vi "Get Logic Statuses.vi"(8 "error in (no error)":errorcluster, 11 "VacuumLine in":refnum<class "VacuumLine.lvclass">) -> (0 "error out":errorcluster, 1 "disconnected":bool, 2 "Array of Logic Statuses":T1(array[cluster]), 3 "VacuumLine out":refnum<class "VacuumLine.lvclass">)   [LabVIEW 2016, in "Hardware.lvlib" / "VacuumLine.lvlib" / "VacuumLine.lvclass"]
uses:
  <userlib>/Common Components/Hardware/Abstract System/VacuumLine/VacuumLine/VacuumLine.lvclass
  <userlib>/Common Components/Hardware/Abstract System/VacuumLine/VacuumLine/VacuumLine.lvclass/VacuumLine.ctl
  <userlib>/Common Components/Hardware/LogicIO/LogicIO/LogicIO.lvclass
  C:/Program Files (x86)/National Instruments/LabVIEW 2016/user.lib/Common Components/Hardware/Abstract Hardware/Hardware.lvclass
  <userlib>/Common Components/Hardware/LogicIO/LogicIO/Get Logic Status (multiple).vi
  <userlib>/Common Components/Hardware/Abstract Hardware/Hardware.lvclass
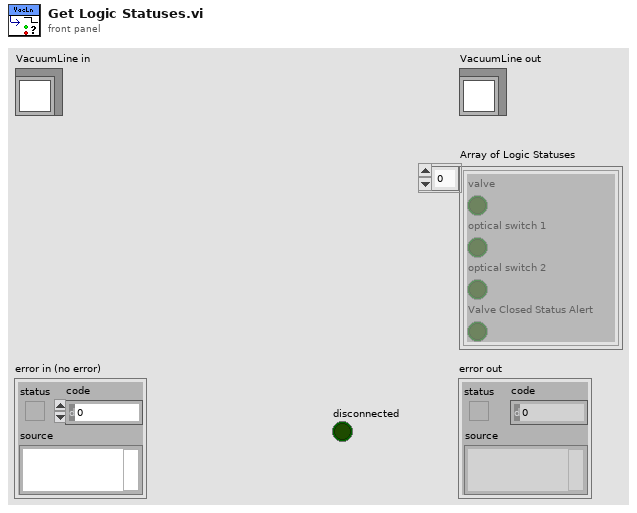
[diagram p1: front panel]
types:
  T1 = cluster{"valve":bool, "optical switch 1":bool, "optical switch 2":bool, "Valve Closed Status Alert":bool}[]
  T2 = cluster{"valve":bool, "optical switch -":bool, "optical switch +":bool, "Valve Closed Status Alert":bool}[]
  T3 = typedef "Hardware.lvlib/VacuumLine.lvlib/VacuumLine.lvclass/Valve Complex.ctl" = cluster{"LogicIO Module":string, "Valve Open":T4, "Optical Switch -":T4, "Optical Switch +":T4, "Valve Closed Status Alert":cluster{"Pin#":u8, "Option":enum16{"Not Used", "Normally Closed"}}}
  T4 = typedef "Hardware.lvlib/VacuumLine.lvlib/VacuumLine.lvclass/Logic Cluster.ctl" = cluster{"Pin#":u8, "Location":dbl, "Tolerance":dbl}
  T5 = cluster{"Array of Logic Statuses[0]":bool, "Array of Logic Statuses[1]":bool, "Array of Logic Statuses[2]":bool, "Array of Logic Statuses[3]":bool}
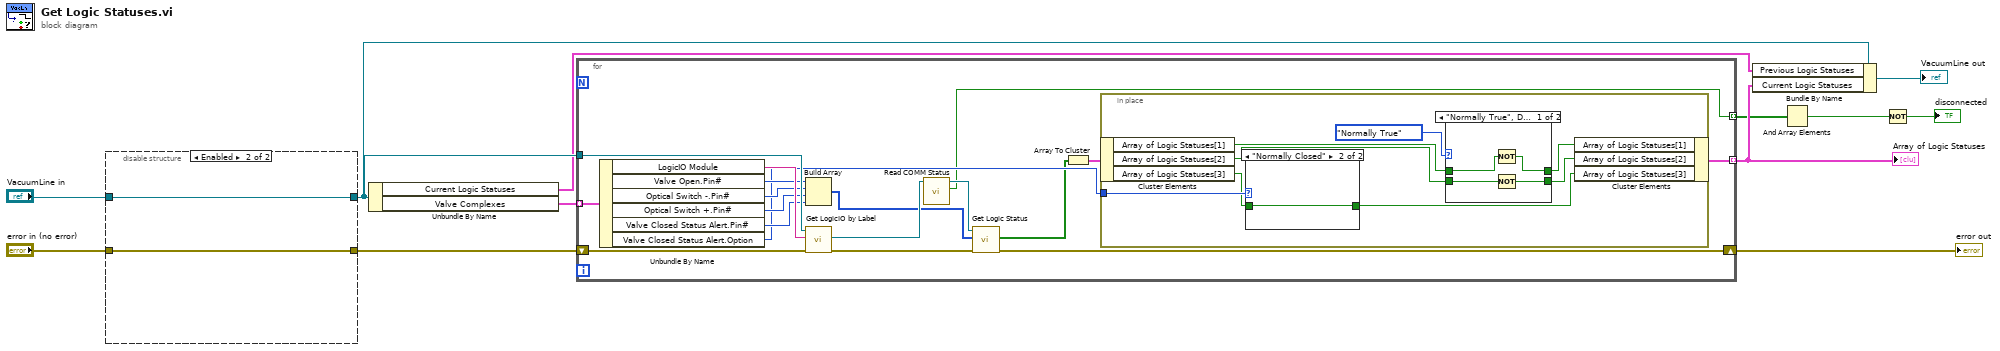
[diagram p0: block diagram]
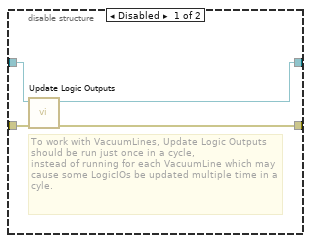
[diagram p2: hidden frame]
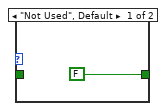
[diagram p3: hidden frame]
diagram:
  n1 = disable-structure shown="Enabled" {
    disable-tunnel: "error in (no error)" -> [w16 w17]
    disable-tunnel: [w15 w17] -> w9
    disable-tunnel: "VacuumLine in" -> [w14 w18]
    disable-tunnel: [w13 w18] -> w7
    frame Disabled {
      # "To work with VacuumLines, Update Logic Outputs should be run just once in a cycle,\ninstead of running for each VacuumLine which may cause some LogicIOs be updated multiple time in a cyle."
      n2 = call <userlib>:"Update Logic Outputs.vi"("error in (no error)"=w16, "VacuumLine in"=w14) -> ("error out"=w15:errorcluster, "VacuumLine out"=w13:refnum<class "VacuumLine.lvclass">)  [unwired: 8 in]
    }
    frame Enabled {
    }
  }
  n3 = Unbundle By Name(w7) -> ("Current Logic Statuses"=w4:T2, "Valve Complexes"=w12:T3[])
  n4 = for {
    tunnel: w12 -> [w36] mode=indexing
    tunnel: w7 -> [w35]
    tunnel: [w25] -> w5 mode=indexing
    shift-right: [w26] -> w10
    shift-left: w9 -> [w28]
    tunnel: [w19] -> w3 mode=indexing
    n5 = Unbundle By Name(w36) -> ("LogicIO Module"=w34:string, "Valve Open.Pin#"=w32:u8, "Optical Switch -.Pin#"=w30:u8, "Optical Switch +.Pin#"=w29:u8, "Valve Closed Status Alert.Pin#"=w24:u8, "Valve Closed Status Alert.Option"=w23:enum16{"Not Used", "Normally Closed"})
    n6 = Build Array(w32, w30, w29, w24) -> (w31:u8[])
    n7 = call <userlib>:"Get LogicIO by Label.vi"("error in (no error)"=w28, "label"=w34, "VacuumLine in"=w35) -> ("error out"=w27:errorcluster, "LogicIO obj"=w33:refnum<class "LogicIO.lvclass">)  [unwired: 5 in, 2 out]
    n8 = call <userlib>:"Read COMM Status.vi"("Hardware in"=w33) -> ("COMM status"=w19:bool, "Hardware out"=w22:refnum<class "LogicIO.lvclass">)  [unwired: 8 in, 1 out]
    n9 = call-poly <userlib>:"Get Logic Status.vi"("error in (no error)"=w27, "Array of Pin #"=w31, "LogicIO in"=w22) -> ("error out"=w26:errorcluster, "Array of Logic Statuses"=w21:bool[])  [unwired: 6 in, 1 out]
    n10 = Array To Cluster(array=w21) -> (cluster=w20:T5)
    n11 = in-place {
      in-place-border: w23 -> [w39]
      n12 = in-place-cluster #1(w20) -> ("Array of Logic Statuses[1]"=w43:bool, "Array of Logic Statuses[2]"=w41:bool, "Array of Logic Statuses[3]"=w37:bool)
      n13 = case shown="\"Normally Closed\"" w39 {
        tunnel: [FALSE w46] -> w38
        tunnel: w37 -> [_ w46]
        frame "Not Used", Default {
        }
        frame "Normally Closed" {
        }
      }
      n14 = case shown="\"Normally True\", Default" enum16{"Normally True", "Normally False"}."Normally True" ("Mode") {
        tunnel: w43 -> [w50 w52]
        tunnel: [w48 w52] -> w42
        tunnel: w41 -> [w49 w51]
        tunnel: [w47 w51] -> w40
        frame "Normally True", Default {
          n15 = Not(x=w50) -> (.not. x?=w48:bool)
          n16 = Not(x=w49) -> (.not. x?=w47:bool)
        }
        frame "Normally False" {
        }
      }
      n17 = in-place-cluster #1("Array of Logic Statuses[1]"=w42, "Array of Logic Statuses[2]"=w40, "Array of Logic Statuses[3]"=w38) -> (w25:T5)
    }
  }
  "error out" <- w10
  "Array of Logic Statuses" <- w5
  n18 = Bundle By Name(cluster=w7, "Previous Logic Statuses"=w4, "Current Logic Statuses"=w5) -> (→"VacuumLine out":refnum<class "VacuumLine.lvclass">)
  n19 = And Array Elements(Boolean array=w3) -> (logical AND=w2:bool)
  n20 = Not(x=w2) -> (.not. x?=→"disconnected":bool)
